vi "ModeEditMain.vi"(0 "当前零件序号":i32) -> (1 "ModelEditInfo":T2, 2 "产品程式设定OK":bool)   [LabVIEW 2014]
uses:
  Global.vi
  <vilib>/Utility/file.llb/Write To Spreadsheet File (I64).vi
  ModeEditeControl.ctl
  ModelInfo.ctl
  Controls/XYZRPos.ctl
panel:
  in  "托盘1螺丝型号":T1=enum."一字螺丝M2.5*8"
  in  "Btn_添加点位":bool
  in  "Btn_删除点位":bool
  in  "退出按钮":bool
  in  "选项卡控件":enum32{"产品程式维护", "锁螺丝点位维护", "点位示意图", "拧紧程式参数维护"}(tab)
  out "已建立产品程式信息":string[][](table)=[["产品型号1", "0", "5", "6", "E:\\771半自动装配系统-2019200427\\Model\\产品型号1\\产品型号1_CAD点位坐标.txt", "0", "0", "0", "0", "0", "0", "0", "1", "92", "93", "93", "94", "95", "94", "97", "94", "92", "93", "18500", "18500"]]
  out "提示信息":string
  in  "Btn_添加新产品程式":bool
  in  "Btn_删除产品程式":bool
  in  "Btn_更新产品程式信息":bool
  in  "产品信息":T3
  in  "Btn_PCB2~4锁螺丝时机械手角度，取料托盘号与PCB1相同":bool
  out "Mark拍照点坐标":T4[](array[typedef])
  in  "Btn_读取Mark1&Mark2(P21 P22)坐标":bool
  in  "Btn_根据第1组Mark点计算PCB1其它拍照点坐标":bool
  in  "读取CAD文档点位信息":bool
  in  "Btn_更新点位信息表":bool
  out "实际点位示意图":T6(plugin-control)
  out "CAD图纸点位示意图":T6(plugin-control)
  in  "Btn_删除拧紧程式参数":bool
  in  "Btn_更新拧紧程式参数":bool
  in  "拧紧程式参数表":string[][](table)=[["92", "2", "3", "4", "6", "7", "8", "9"], ["93", "12", "13", "14", "16", "17", "18", "19"], ["94", "22", "23", "24", "26", "27", "28", "29"], ["95", "32", "33", "34", "36", "37", "38", "39"]]
  out "不同型号螺丝放料点与拍照点高度差":string[][](table)=[["一字螺丝M2.5*4"], ["一字螺丝M2.5*6"], ["一字螺丝M2.5*8"], ["一字螺丝M2.5*10"], ["一字螺丝M2.5*12"], ["一字螺丝M2.5*14"], ["一字螺丝M2.5*16"], ["一字螺丝M2.5*18"], ["一字螺丝M2.5*20"], ["一字螺丝M3*4"], ["一字螺丝M3*6"], ["一字螺丝M3*8"], ["一字螺丝M3*10"], ["一字螺丝M3*12"], ["一字螺丝M3*14"], ["一字螺丝M3*16"], ["一字螺丝M3*18"], ["一字螺丝M3*20"], ["一字螺丝M4*6"], ["一字螺丝M4*8"], ["一字螺丝M4*10"], ["一字螺丝M4*12"], ["一字螺丝M4*14"], ["一字螺丝M4*16"], ["一字螺丝M4*18"], ["一字螺丝M4*20"], ["十字螺丝M2.5*4"], ["十字螺丝M2.5*6"], ["十字螺丝M2.5*8"], ["十字螺丝M2.5*10"], ["十字螺丝M2.5*12"], ["十字螺丝M2.5*14"], ["十字螺丝M2.5*16"], ["十字螺丝M2.5*18"], ["十字螺丝M2.5*20"], ["十字螺丝M3*4"], ["十字螺丝M3*6"], ["十字螺丝M3*8"], ["十字螺丝M3*10"], ["十字螺丝M3*12"], ["十字螺丝M3*14"], ["十字螺丝M3*16"], ["十字螺丝M3*18"], ["十字螺丝M3*20"], ["十字螺丝M4*6"], ["十字螺丝M4*8"], ["十字螺丝M4*10"], ["十字螺丝M4*12"], ["十字螺丝M4*14"], ["十字螺丝M4*16"], ["十字螺丝M4*18"], ["十字螺丝M4*20"]]
  # "白色代表自动锁螺丝，灰色不锁"
  # "白色代表自动锁螺丝，灰色不锁"
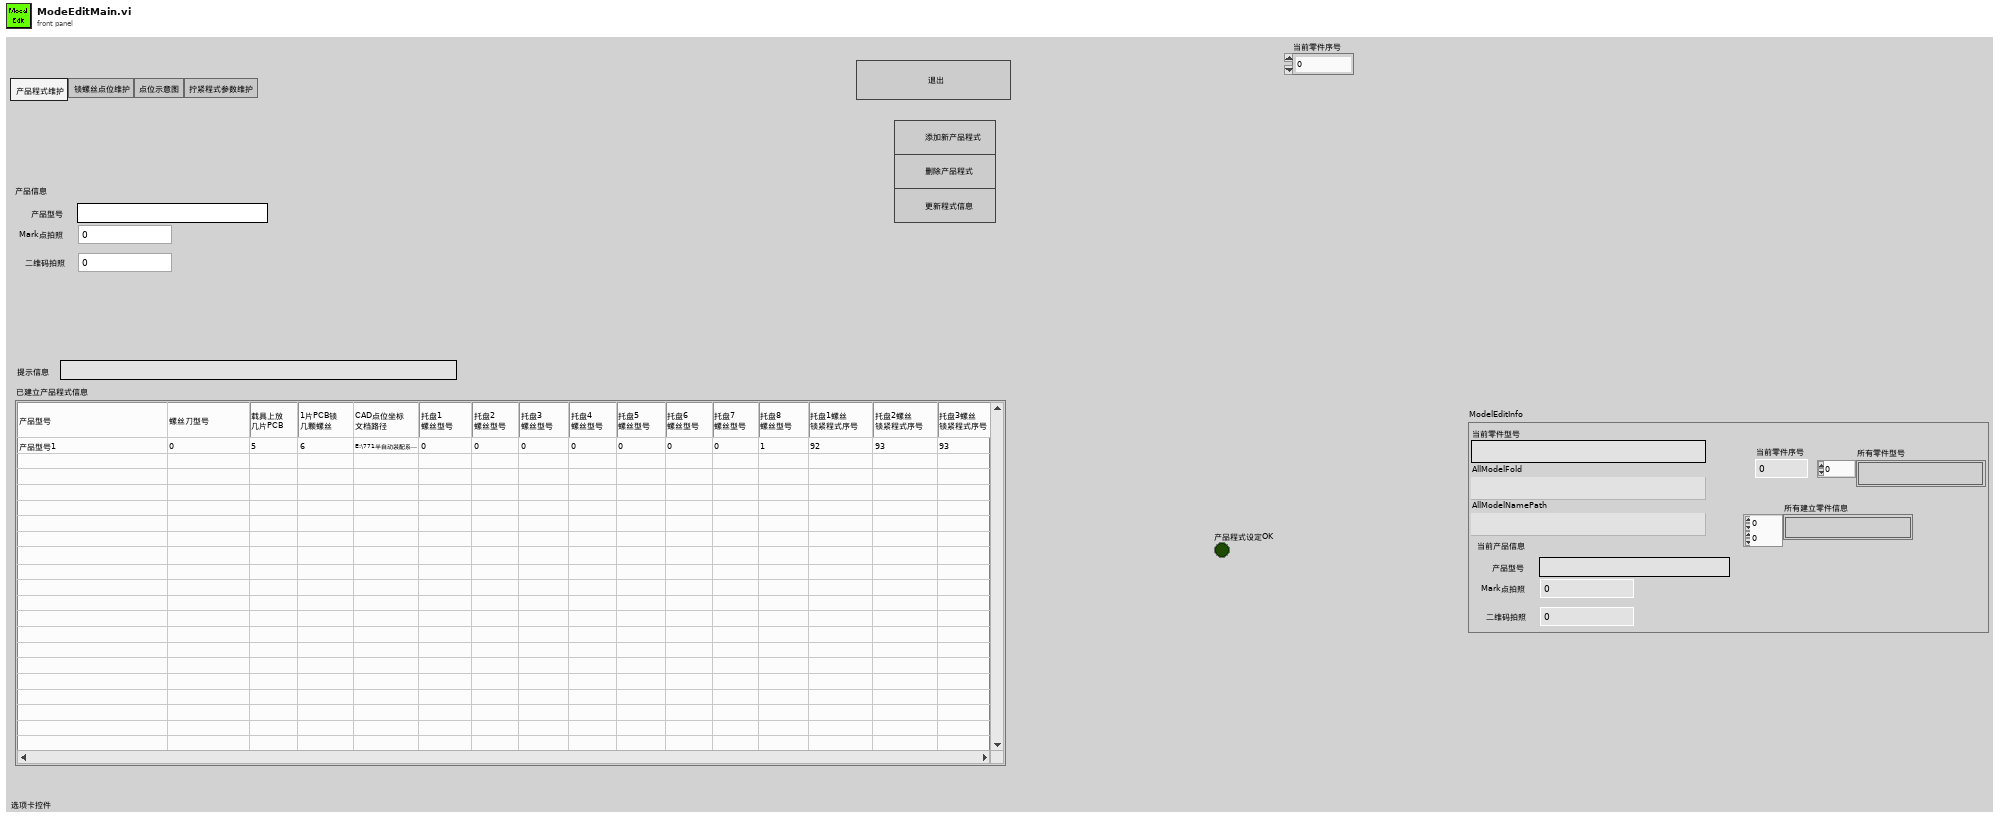
[diagram p1: front panel]
types:
  T1 = typedef "控件-螺丝型号.ctl" = enum16{"不供料", "一字螺丝M2.5*4", "一字螺丝M2.5*6", "一字螺丝M2.5*8", "一字螺丝M2.5*10", "一字螺丝M2.5*12", "一字螺丝M2.5*14", "一字螺丝M2.5*16", "一字螺丝M2.5*18", "一字螺丝M2.5*20", "一字螺丝M3*4", "一字螺丝M3*6", "一字螺丝M3*8", "一字螺丝M3*10", "一字螺丝M3*12", "一字螺丝M3*14", "一字螺丝M3*16", "一字螺丝M3*18", "一字螺丝M3*20", "一字螺丝M4*6", "一字螺丝M4*8", "一字螺丝M4*10", "一字螺丝M4*12", "一字螺丝M4*14", "一字螺丝M4*16", "一字螺丝M4*18", "一字螺丝M4*20", "十字螺丝M2.5*4", "十字螺丝M2.5*6", "十字螺丝M2.5*8", "十字螺丝M2.5*10", "十字螺丝M2.5*12", "十字螺丝M2.5*14", "十字螺丝M2.5*16", "十字螺丝M2.5*18", "十字螺丝M2.5*20", "十字螺丝M3*4", "十字螺丝M3*6", "十字螺丝M3*8", "十字螺丝M3*10", "十字螺丝M3*12", "十字螺丝M3*14", "十字螺丝M3*16", "十字螺丝M3*18", "十字螺丝M3*20", "十字螺丝M4*6", "十字螺丝M4*8", "十字螺丝M4*10", "十字螺丝M4*12", "十字螺丝M4*14", "十字螺丝M4*16", "十字螺丝M4*18", "十字螺丝M4*20"}
  T2 = typedef "ModeEditeControl.ctl" = cluster{"AllModelFold":path, "AllModelNamePath":path, "所有零件型号":string[], "当前零件型号":string, "所有建立零件信息":string[][], "当前零件序号":i32, "当前产品信息":T3}
  T3 = typedef "ModelInfo.ctl" = cluster{"产品型号":string, "二维码拍照":u32, "Mark点拍照":u32}
  T4 = typedef "XYZRPos+左右手.ctl" = cluster{"坐标":T5, "左右手":dbl}
  T5 = typedef "XYZRPos.ctl" = cluster{"X":dbl, "Y":dbl, "Z":dbl, "R":dbl}
  T6 = typedef "IMAQ Image.ctl" = refnum<image>
  T7 = typedef "控件-点位示意图动作.ctl" = enum16{"初始化点位示意图", "更新点位示意图"}
  T8 = cluster{"CAD图纸点位示意图":refnum<vi>, "实际点位示意图":refnum<vi>}
  T9 = typedef "ModeEditeControl.ctl" = cluster{"Root":path, "AllModelFold":path, "AllModelNamePath":path, "所有零件型号":string[], "当前零件型号":string, "所有建立零件信息":string[][], "当前零件序号":i32, "当前产品所有点位信息":cluster{"当前点位序号":i32, "点位信息路径":path, "CAD点位坐标路径":path, "点位信息表":string[][], "当前点位信息":T10, "CAD图纸点位个数":i32}, "当前产品信息":T13, "所有螺丝和垫片型号Path":path, "Mark拍照点坐标":T4[][], "自动锁螺丝: PCB孔拍照点-多片PCB(去除未勾选的)":T4[], "8个供料盘是否供料-1PCB(去除未勾选的)":bool[], "8个供料盘是否拍照取料":bool[], "自动锁螺丝: 1PCB每颗螺丝来自哪个供料盘U8(去除未勾选的)":u8[], "自动锁螺丝: 1PCB每颗螺丝拧紧程式编号U8(去除未勾选的)":u8[], "4个预锁程式+4个复锁程式编号U8":u8[], "自动锁螺丝: 锁螺丝相对拍照时旋转角度-多片PCB(去除未勾选的)":i32[], "自动锁螺丝: 点位补偿值-多片PCB(去除未勾选的)":T11[], "1PCB上自动锁螺丝个数(去除未勾选的)":i32, "自动锁螺丝: 放料点相对拍照点高度差-多片PCB(去除未勾选的)":dbl[], "8个供料盘是否供料(包括未勾选的)":bool[], "已勾选的自动锁螺丝点位供料盘设定错误":bool, "自动锁螺丝: 复锁拍照点-多片PCB(去除未勾选的)":T4[][], "自动锁螺丝: 1PCB每颗螺丝外径*10(去除未勾选的)":u32[], "拧紧程式参数":cluster{"所有拧紧程式参数表路径":path, "所有拧紧程式参数表":string[][], "自动锁螺丝: 每个托盘螺丝拧紧程式参数":T15[], "自动锁螺丝: 预锁复锁拧紧程式参数":T15[], "所有拧紧程式参数表当前行":i32}, "已勾选的自动锁螺丝点位拧紧程式序号设定错误":bool}
  T10 = typedef "锁附点位信息.ctl" = cluster{"点位名称":string, "点位坐标(图纸)":T11, "点位坐标(实际)":T5, "补偿值":T11, "锁附时机械手角度":T12, "放料点相对Mark\n拍照点高度差":dbl, "选择螺丝托盘":enum32{"托盘1", "托盘2", "托盘3", "托盘4", "托盘5", "托盘6", "托盘7", "托盘8"}, "拧紧程式序号":u16, "预锁程式序号":u16, "复锁程式序号":u16, "自动锁螺丝":bool}
  T11 = typedef "XYZPos.ctl" = cluster{"X":dbl, "Y":dbl, "Z":dbl}
  T12 = typedef "锁附时机械手角度.ctl" = enum16{"0度", "顺时针90度", "顺时针180度", "逆时针90度", "逆时针180度"}
  T13 = typedef "ModelInfo.ctl" = cluster{"产品型号":string, "螺丝刀型号":T14, "载具上放几片PCB":u16, "1片PCB锁几颗螺丝":u16, "CAD点位坐标文档路径":path, "托盘1螺丝型号":T1, "托盘2螺丝型号":T1, "托盘3螺丝型号":T1, "托盘4螺丝型号":T1, "托盘5螺丝型号":T1, "托盘6螺丝型号":T1, "托盘7螺丝型号":T1, "托盘8螺丝型号":T1, "托盘1螺丝锁紧程式序号":u32, "托盘2螺丝锁紧程式序号":u32, "托盘3螺丝锁紧程式序号":u32, "托盘4螺丝锁紧程式序号":u32, "托盘5螺丝锁紧程式序号":u32, "托盘6螺丝锁紧程式序号":u32, "托盘7螺丝锁紧程式序号":u32, "托盘8螺丝锁紧程式序号":u32, "预锁程式序号":u32, "复锁程式序号":u32, "复锁拍照点与Mark拍照点高度差":dbl, "取料点与P2高度差":dbl, "拍PCB孔曝光时间":u32, "取料拍螺帽曝光时间":u32, "复锁拍螺帽曝光时间":u32, "下相机曝光时间":u32}
  T14 = typedef "螺丝刀类型.ctl" = enum16{"螺丝刀1-1*3mm", "螺丝刀2-1.5*3mm", "螺丝刀3-2*3mm", "螺丝刀4-2*4mm", "螺丝刀5-2.5*4mm"}
  T15 = typedef "控件-拧紧程式参数.ctl" = cluster{"螺距":dbl, "入牙段转速":dbl, "入牙段转角":dbl, "快速段转速":dbl, "快速段转角":dbl, "快速段Z补偿":dbl, "拧紧转速":dbl}
  T16 = typedef "欧姆龙PLC Action.ctl" = enum16{"读设备状态", "初始化", "待命", "重新初始化", "读触发信息", "读第1组Mark点坐标", "读第2组Mark点坐标", "写基本信息", "写第1组Mark点坐标", "写第2组Mark点坐标", "写相机中心到出线头的距离", "写一笔轨迹到PLC", "写入进线前段点位", "写入板内布线点位", "写入出线布线点位", "写入数据写入完成信号", "获取信息", "写入进出线方向", "写加工信号"}
  T17 = typedef "欧姆龙PLC Action.ctl" = enum16{"初始化", "重新初始化", "读触发信息", "读示教坐标P1P2", "读示教坐标P3P4", "读示教坐标P11P12", "读示教坐标P13P14", "读第1组Mark点坐标", "读第2组Mark点坐标", "读第3组Mark点坐标", "自检：写螺丝刀拍照结果和Finish", "自检：写供料盘二维码拍照结果和Finish", "读第4组Mark点坐标", "写取料点相对拍照点移动量", "写放料点坐标", "写放螺丝时相对当前拍照点偏移量", "写取料点相对拍照点移动量&放料点坐标", "写螺杆拍照完成Finish", "写读取锁附结果完成信号", "写复锁时相对拍照点移动量", "写数据-测试用", "写当前产品基本供料信息", "写当前产品每颗螺丝来自哪个供料盘", "写当前产品每颗螺丝拧紧程式序号", "写当前产品4个预锁程式和4个复锁程式序号", "写第1组Mark点坐标", "写第2组Mark点坐标", "写第3组Mark点坐标", "写第4组Mark点坐标", "写夹螺杆点到拍螺帽点距离", "写第1组复锁拍照点", "写第2组复锁拍照点", "写第3组复锁拍照点", "写第4组复锁拍照点", "写启用的托盘螺丝拧紧程式参数", "写预锁复锁拧紧程式参数", "获取信息"}
  T18 = enum16{"计算PCB1其它拍照点坐标", "计算PCB2其它拍照点坐标", "计算PCB3其它拍照点坐标", "计算PCB4其它拍照点坐标"}
  T19 = typedef "LVRowAndColumnTypeDef.ctl" = cluster{"Row":i32, "Column":i32}
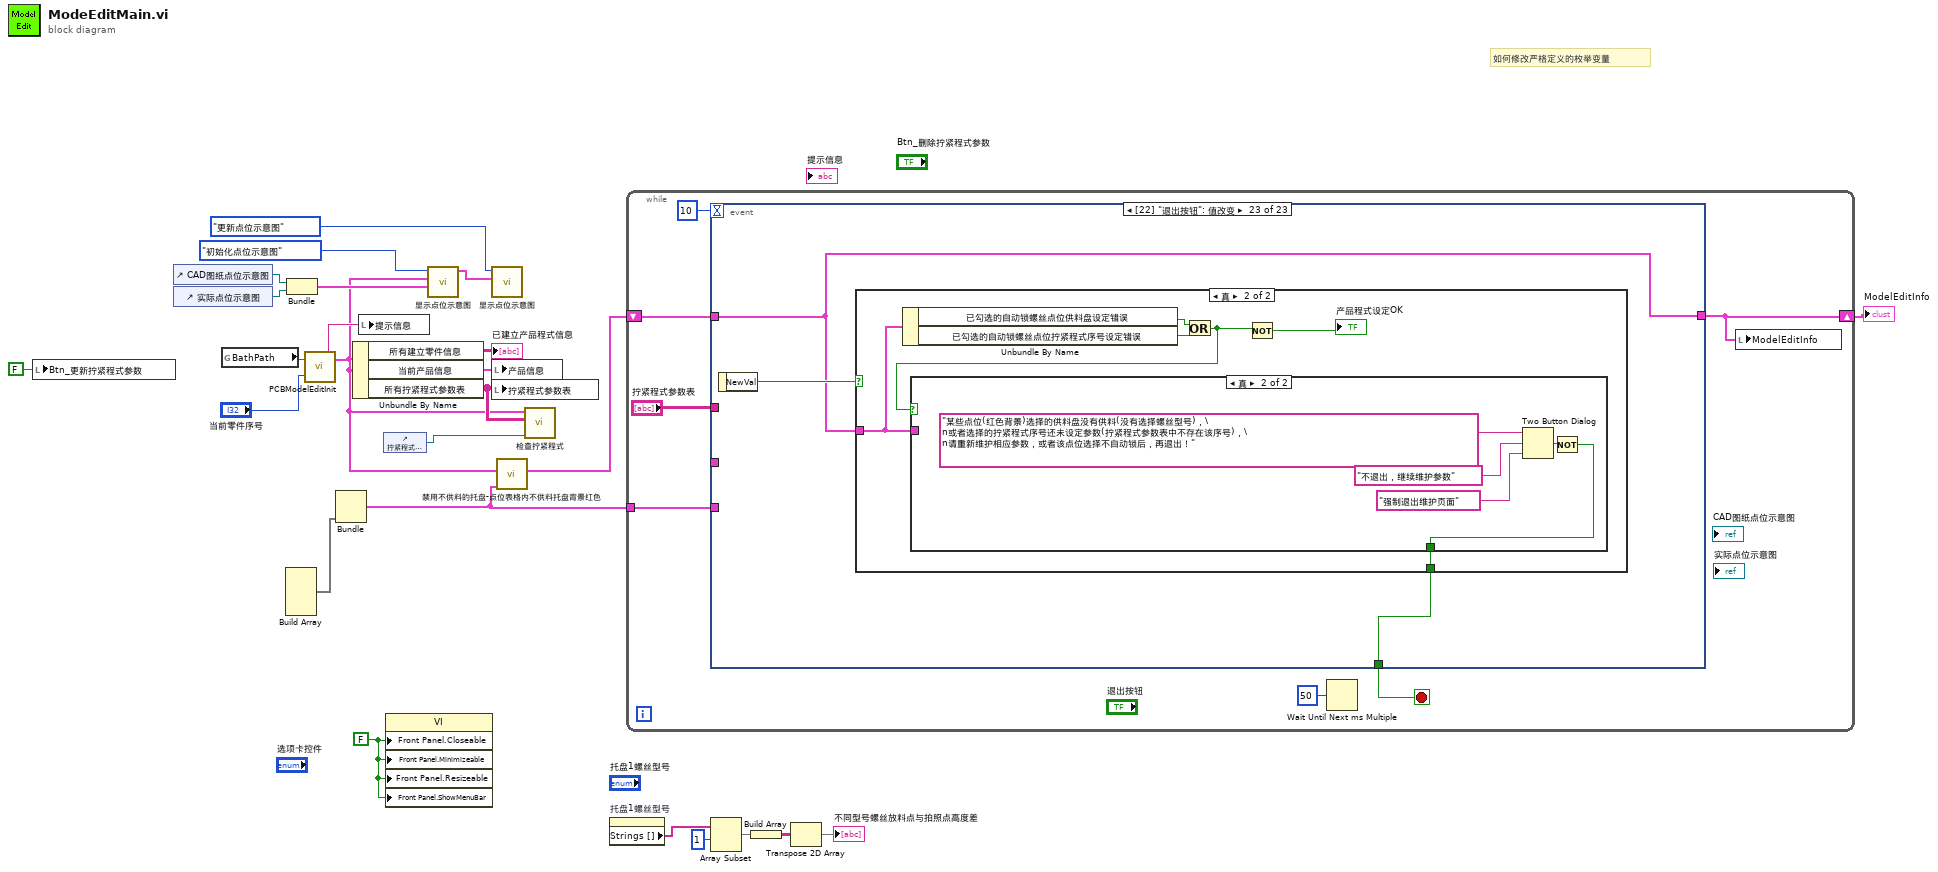
[diagram p0: block diagram]
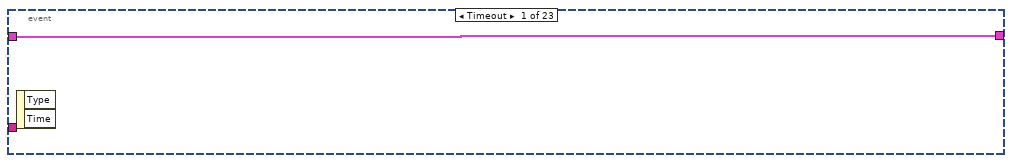
[diagram p2: hidden frame]
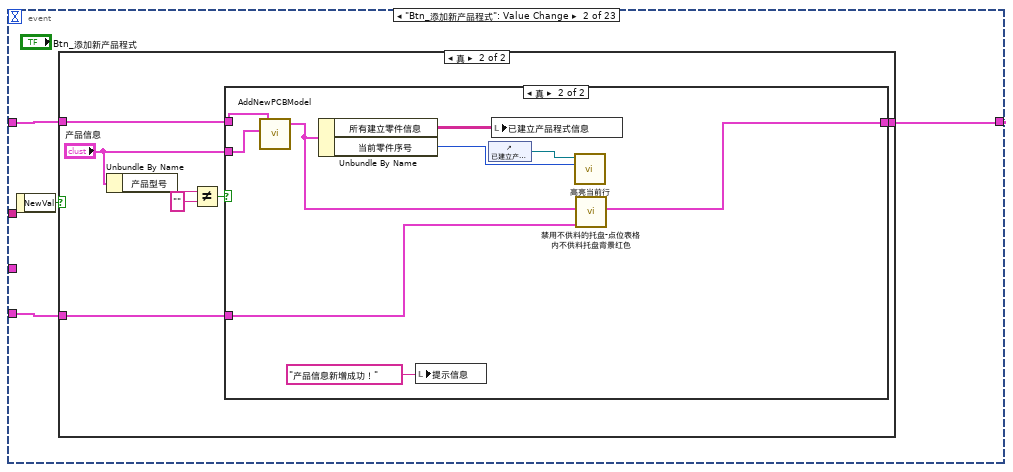
[diagram p3: hidden frame]
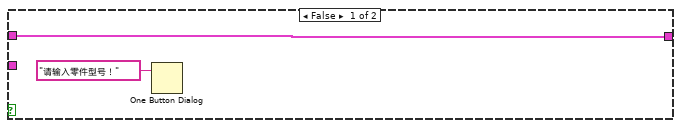
[diagram p5: hidden frame]
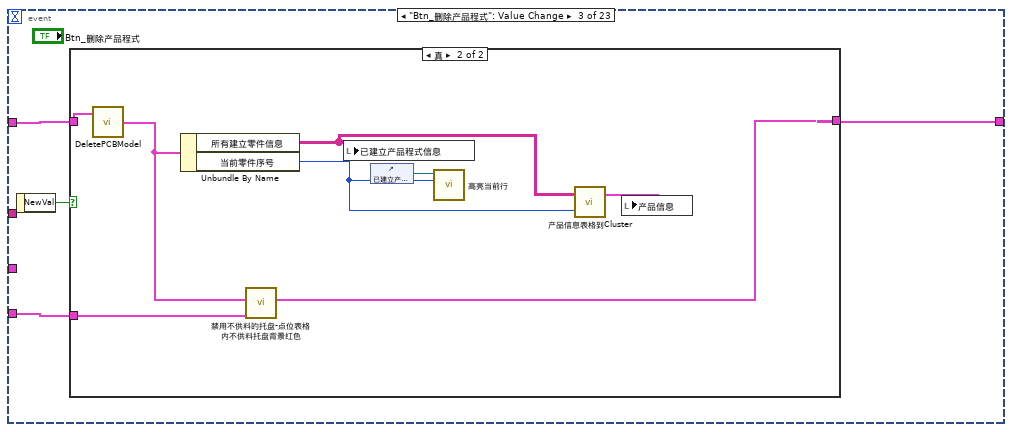
[diagram p6: hidden frame]
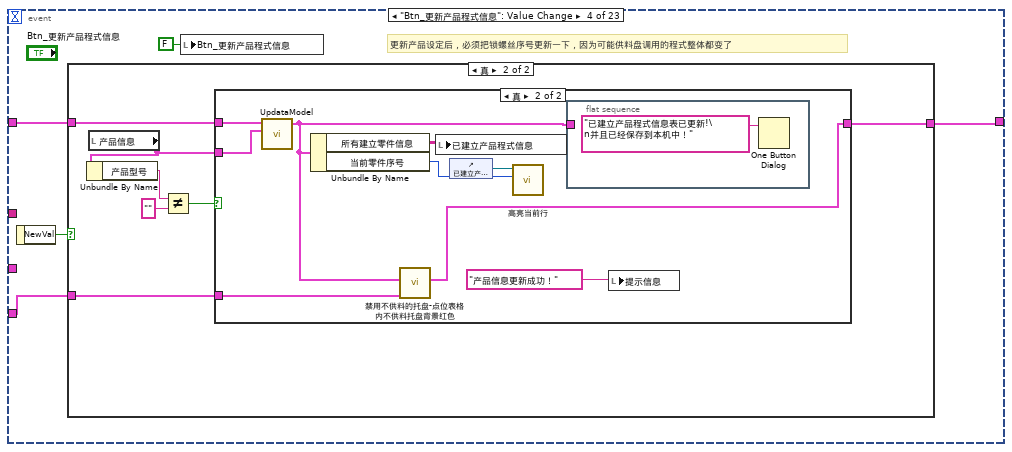
[diagram p8: hidden frame]
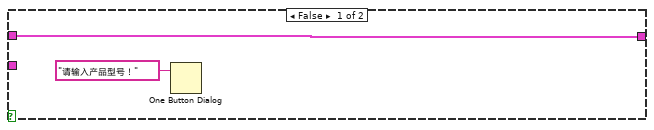
[diagram p10: hidden frame]
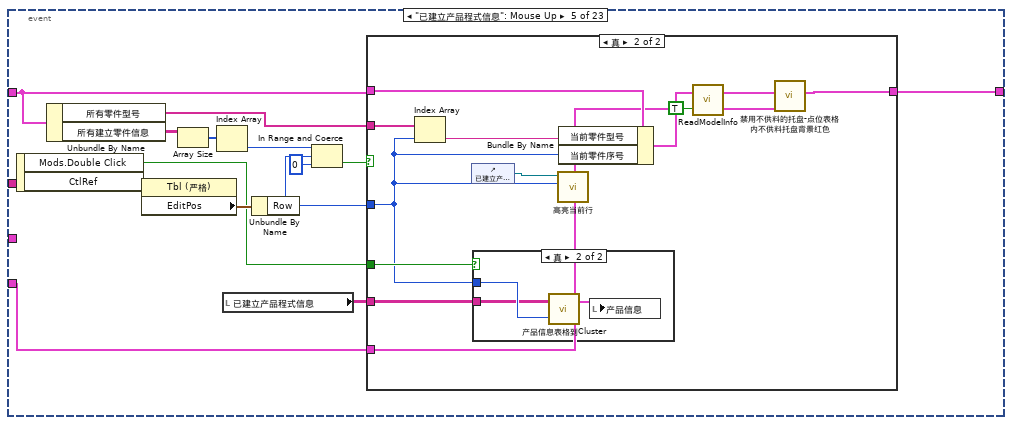
[diagram p11: hidden frame]
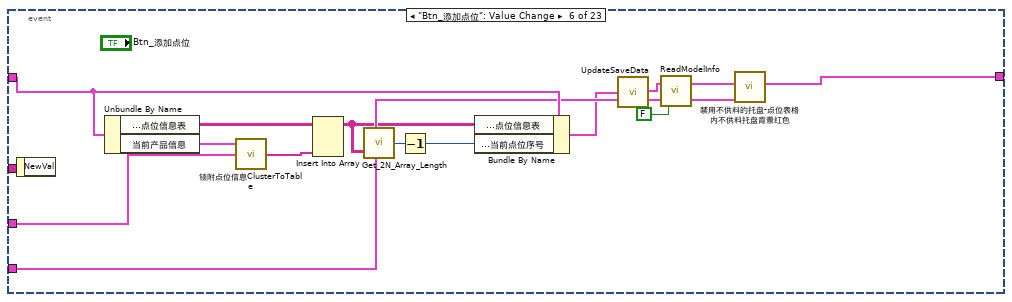
[diagram p14: hidden frame]
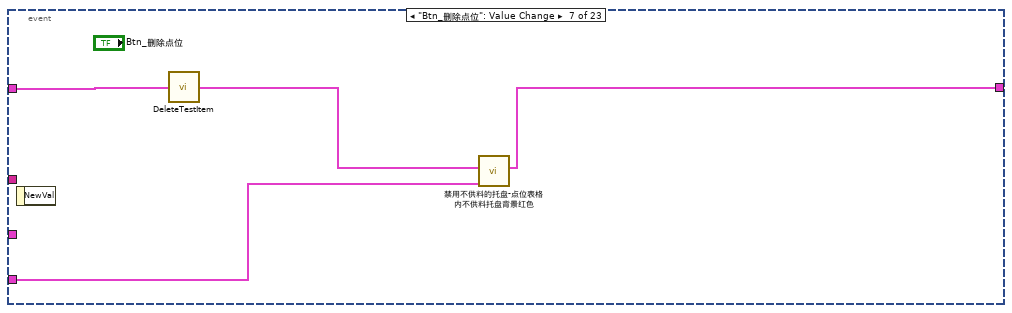
[diagram p15: hidden frame]
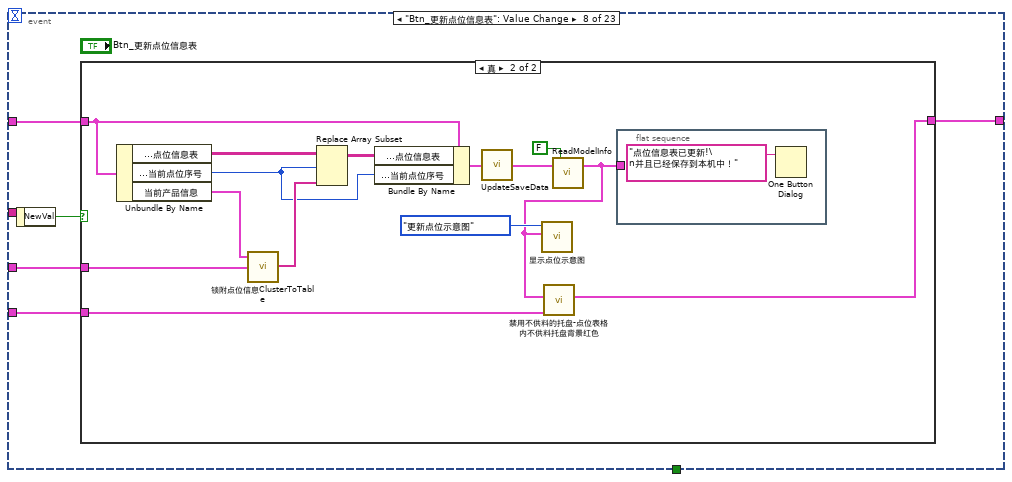
[diagram p16: hidden frame]
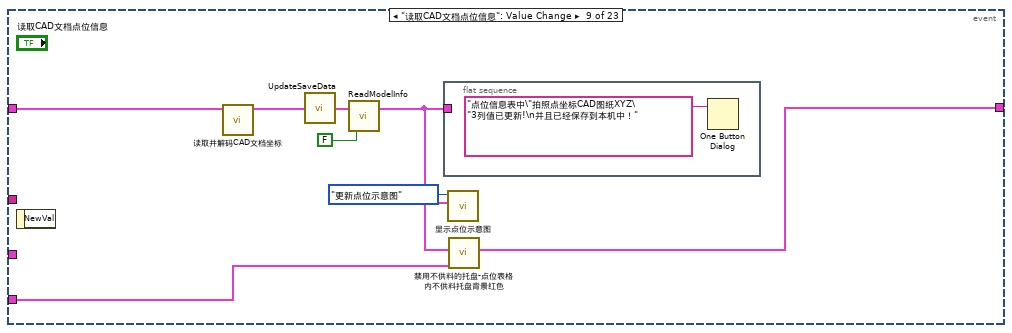
[diagram p18: hidden frame]
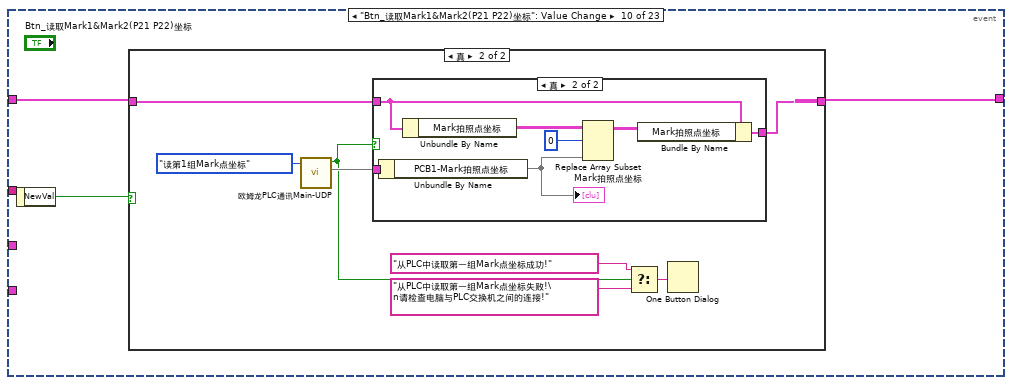
[diagram p19: hidden frame]
diagram:
  w30 = FALSE ("Front Panel Window:Closeable")
  # "如何修改严格定义的枚举变量"
  n1 = local write "Btn_更新拧紧程式参数"(FALSE ("Btn_更新拧紧程式参数")) -> ()
  n2 = control-ref of="CAD图纸点位示意图"() -> (w25:refnum<vi>)
  n3 = control-ref of="实际点位示意图"() -> (w24:refnum<vi>)
  n4 = global read "Global.vi" "BathPath"() -> (w32:path)
  n5 = Build Array() -> (w13:void[], w19:dbl, w18:dbl, w17:dbl, w16:dbl, w15:dbl, w14:dbl)
  n6 = Bundle("CAD图纸点位示意图"=w25, "实际点位示意图"=w24) -> (w23:T8)  [unwired: 1 in]
  n7 = call "PCBModelEditInit.vi"("当前零件序号"="当前零件序号", "path"=w32) -> ("Msg"=w31:string, "ModelEditInfo"=w2:T2)
  n8 = Bundle(w13) -> (w11:cluster{void, void, void, void[]}, w12, w27)  [unwired: 2 in]
  n9 = Unbundle By Name(w2) -> ("所有建立零件信息"=→"已建立产品程式信息":string[][], "当前产品信息"=w26:T3, "所有拧紧程式参数表"=w3:string[][])
  n10 = local write "提示信息"(w31) -> ()
  n11 = control-ref of="拧紧程式参数表"() -> (w1:refnum<vi>)
  n12 = property class="VI"("Front Panel.Closeable"=w30, "Front Panel.Minimizeable"=w30, "Front Panel.Resizeable"=w30, "Front Panel.ShowMenuBar"=w30) -> ()  [unwired: 2 in, 2 out]
  n13 = call "显示点位示意图.vi"("Img引用Cluster"=w23, "ModelEditInfo"=w2, "显示点位动作"=控件-点位示意图动作."初始化点位示意图") -> ("ModelEditInfo out"=w20:T2)  [unwired: 8 in]
  n14 = call "显示点位示意图.vi"("ModelEditInfo"=w20, "显示点位动作"=控件-点位示意图动作."更新点位示意图") -> ()  [unwired: 9 in, 1 out]
  n15 = local write "产品信息"(w26) -> ()
  n16 = local write "拧紧程式参数表"(w3) -> ()
  n17 = call "禁用不供料的托盘-点位表格内不供料托盘背景红色.vi"("引用Cluster"=w11, "ModelEditInfo in"=w2) -> ("ModelEditInfo out"=w10:T9)  [unwired: 8 in, 1 out]
  n18 = call "检查拧紧程式.vi"("拧紧程式参数表引用"=w1, "拧紧程式参数表输入"=w3, "ModelEditInfo"=w2) -> ()  [unwired: 7 in, 2 out]
  n19 = property on="托盘1螺丝型号" class="Enum (严格)"() -> ("Strings []"=w9:string[])  [unwired: 2 in, 2 out]
  n20 = while {
    shift-right: [w36] -> w33
    shift-left: w10 -> [w39]
    tunnel: w11 -> [w35]
    stop <- w38 stop-if-true
    n21 = event shown="[22] \"退出按钮\": 值改变" {
      selector: _ -> [_ _ _ _ _ _ _ _ _ _ _ _ _ _ _ _ _ _ _ _ _ _ _]
      dyn-events: _ -> [_ _ _ _ _ _ _ _ _ _ _ _ _ _ _ _ _ _ _ _ _ _ _]
      timeout: 10 -> [_ _ _ _ _ _ _ _ _ _ _ _ _ _ _ _ _ _ _ _ _ _ _]
      tunnel: w39 -> [w42 w45 w68 w83 w109 w145 w151 w155 w180 w184 w203 w224 w244 w270 w278 w288 w298 w308 w315 w341 w379 w383 w400]
      tunnel: [w42 w44 w67 w82 w108 w134 w148 w153 w173 w182 w202 w222 w242 w262 w272 w283 w292 w302 w314 w346 w373 w386 w400] -> w36
      tunnel: [_ _ _ _ _ _ _ _ _ _ _ _ _ _ _ _ _ _ _ _ _ _ w401] -> w38
      tunnel: [_ _ _ _ _ w144 _ w154 _ _ _ _ _ _ _ _ _ _ _ _ _ _ _] -> w37
      tunnel: w35 -> [_ w43 w66 w79 w104 w141 w149 w152 w176 _ _ _ _ w265 w275 w286 w296 w304 w310 w345 w372 _ _]
      tunnel: "拧紧程式参数表" -> [_ _ _ _ _ _ _ _ _ _ _ _ _ _ _ _ _ _ _ w342 _ _ _]
      event Timeout {
        n22 = event-data() -> ()  [unwired: 1 in, 2 out]
      }
      event "Btn_添加新产品程式": Value Change {
        n23 = event-data() -> ("NewVal"=w46:bool)  [unwired: 1 in]
        n24 = case shown="真" w46 {
          tunnel: w45 -> [w47 w51]
          tunnel: [w47 w52] -> w44
          tunnel: w43 -> [_ w48]
          frame False {
          }
          frame True {
            n25 = Unbundle By Name("产品信息") -> ("产品型号"=w50:string)
            n26 = Not Equal?(x=w50, y="") -> (x != y?=w53:bool)
            n27 = case shown="真" w53 {
              tunnel: w51 -> [w55 w65]
              tunnel: [w55 w57] -> w52
              tunnel: "产品信息" -> [_ w62]
              tunnel: w48 -> [_ w58]
              frame False {
                n28 = One Button Dialog(message="请输入零件型号！") -> ()  [unwired: 1 in, 1 out]
              }
              frame True {
                n29 = call "AddNewPCBModel.vi"("新增零件信息"=w62, "ModelEditInfo in"=w65) -> ("ModelEditInfo out"=w59:T2)  [unwired: 4 in]
                n30 = Unbundle By Name(w59) -> ("所有建立零件信息"=w63:string[][], "当前零件序号"=w60:i32)
                n31 = local write "提示信息"("产品信息新增成功！" ("ReadGerberMsg")) -> ()
                n32 = control-ref of="已建立产品程式信息"() -> (w61:refnum<vi>)
                n33 = local write "已建立产品程式信息"(w63) -> ()
                n34 = call "高亮当前行.vi"("Row"=w60, "Table输入"=w61) -> ()  [unwired: 9 in, 1 out]
                n35 = call "禁用不供料的托盘-点位表格内不供料托盘背景红色.vi"("引用Cluster"=w58, "ModelEditInfo in"=w59) -> ("ModelEditInfo out"=w57:T9)  [unwired: 8 in, 1 out]
              }
            }
          }
        }
      }
      event "Btn_删除产品程式": Value Change {
        n36 = event-data() -> ("NewVal"=w69:bool)  [unwired: 1 in]
        n37 = case shown="真" w69 {
          tunnel: w68 -> [w70 w78]
          tunnel: [w70 w71] -> w67
          tunnel: w66 -> [_ w72]
          frame False {
          }
          frame True {
            n38 = call "DeletePCBModel.vi"("ModelEditInfo in"=w78) -> ("ModelEditInfo out"=w73:T2)
            n39 = Unbundle By Name(w73) -> ("所有建立零件信息"=w75:string[][], "当前零件序号"=w76:i32)
            n40 = call "禁用不供料的托盘-点位表格内不供料托盘背景红色.vi"("引用Cluster"=w72, "ModelEditInfo in"=w73) -> ("ModelEditInfo out"=w71:T9)  [unwired: 8 in, 1 out]
            n41 = local write "已建立产品程式信息"(w75) -> ()
            n42 = control-ref of="已建立产品程式信息"() -> (w77:refnum<vi>)
            n43 = call "高亮当前行.vi"("Row"=w76, "Table输入"=w77) -> ()  [unwired: 9 in, 1 out]
            n44 = call "产品信息表格到Cluster.vi"("Row"=w76, "已建立量测零件信息"=w75) -> ("零件信息"=w74:T13)
            n45 = local write "产品信息"(w74) -> ()
          }
        }
      }
      event "Btn_更新产品程式信息": Value Change {
        # "更新产品设定后，必须把锁螺丝序号更新一下，因为可能供料盘调用的程式整体都变了"
        n46 = event-data() -> ("NewVal"=w81:bool)  [unwired: 1 in]
        n47 = case shown="真" w81 {
          tunnel: w83 -> [w84 w88]
          tunnel: [w84 w87] -> w82
          tunnel: w79 -> [_ w85]
          frame False {
          }
          frame True {
            n48 = local read "产品信息"() -> (w86:T3)
            n49 = Unbundle By Name(w86) -> ("产品型号"=w89:string)
            n50 = Not Equal?(x=w89, y="") -> (x != y?=w90:bool)
            n51 = case shown="真" w90 {
              tunnel: w88 -> [w92 w100]
              tunnel: [w92 w94] -> w87
              tunnel: w86 -> [_ w99]
              tunnel: w85 -> [_ w96]
              frame False {
                n52 = One Button Dialog(message="请输入产品型号！") -> ()  [unwired: 1 in, 1 out]
              }
              frame True {
                n53 = call "UpdataModel.vi"("更新零件信息"=w99, "ModelEditInfo in"=w100) -> ("ModelEditInfo out"=w95:T2)  [unwired: 4 in]
                n54 = Unbundle By Name(w95) -> ("所有建立零件信息"=w102:string[][], "当前零件序号"=w97:i32)
                n55 = call "禁用不供料的托盘-点位表格内不供料托盘背景红色.vi"("引用Cluster"=w96, "ModelEditInfo in"=w95) -> ("ModelEditInfo out"=w94:T9)  [unwired: 8 in, 1 out]
                n56 = local write "已建立产品程式信息"(w102) -> ()
                n57 = control-ref of="已建立产品程式信息"() -> (w98:refnum<vi>)
                n58 = call "高亮当前行.vi"("Row"=w97, "Table输入"=w98) -> ()  [unwired: 9 in, 1 out]
                n59 = flat-sequence {
                  tunnel: w95 -> [_]
                  frame #0 {
                    n60 = One Button Dialog(message="已建立产品程式信息表已更新!\n并且已经保存到本机中！" ("消息")) -> ()  [unwired: 1 in, 1 out]
                  }
                }
                n61 = local write "提示信息"("产品信息更新成功！" ("ReadGerberMsg")) -> ()
              }
            }
          }
        }
        n62 = local write "Btn_更新产品程式信息"(FALSE ("Btn_更新量测信息")) -> ()
      }
      event "已建立产品程式信息": Mouse Up {
        n63 = event-data() -> ("Mods.Double Click"=w106:bool, "CtlRef"=w116:refnum<vi>)  [unwired: 1 in]
        n64 = Unbundle By Name(w109) -> ("所有零件型号"=w107:string[], "所有建立零件信息"=w115:string[][])
        n65 = property class="Tbl (严格)"(reference=w116) -> ("EditPos"=w117:T19)  [unwired: 1 in, 2 out]
        n66 = Array Size(array=w115) -> (size(s)=w114:i32[])
        n67 = Index Array(array=w114) -> (element=w110:i32)  [unwired: 1 in]
        n68 = local read "已建立产品程式信息"() -> (w105:string[][])
        n69 = Unbundle By Name(w117) -> ("Row"=w113:i32)
        n70 = In Range and Coerce(upper limit=w110, x=w113, lower limit=0 ("下限")) -> (In Range?=w112:bool)  [unwired: 1 out]
        n71 = case shown="真" w112 {
          tunnel: w113 -> [_ w123]
          tunnel: w109 -> [w118 w130]
          tunnel: [w118 w119] -> w108
          tunnel: w107 -> [_ w127]
          tunnel: w106 -> [_ w126]
          tunnel: w105 -> [_ w125]
          tunnel: w104 -> [_ w120]
          frame False {
          }
          frame True {
            n72 = Index Array(array=w127, index=w123) -> (element=w129:string)
            n73 = control-ref of="已建立产品程式信息"() -> (w124:refnum<vi>)
            n74 = case shown="真" w126 {
              tunnel: w123 -> [_ w132]
              tunnel: w125 -> [_ w131]
              frame False {
              }
              frame True {
                n75 = call "产品信息表格到Cluster.vi"("Row"=w132, "已建立量测零件信息"=w131) -> ("零件信息"=w133:T13)
                n76 = local write "产品信息"(w133) -> ()
              }
            }
            n77 = call "高亮当前行.vi"("Row"=w123, "Table输入"=w124) -> ()  [unwired: 9 in, 1 out]
            n78 = Bundle By Name(cluster=w130, "当前零件型号"=w129, "当前零件序号"=w123) -> (w128:T9)
            n79 = call "ReadModelInfo.vi"("更新量测项目序号"=TRUE, "ModelEditInfo in"=w128) -> ("ModelEditInfo out"=w121:T2)  [unwired: 1 in]
            n80 = call "禁用不供料的托盘-点位表格内不供料托盘背景红色.vi"("引用Cluster"=w120, "ModelEditInfo in"=w121) -> ("ModelEditInfo out"=w119:T9)  [unwired: 8 in, 1 out]
          }
        }
      }
      event "Btn_添加点位": Value Change {
        n81 = event-data() -> ()  [unwired: 1 in, 1 out]
        n82 = Unbundle By Name(w145) -> ("当前产品所有点位信息.点位信息表"=w146:string[][], "当前产品信息"=w142:T13)
        n83 = call "锁附点位信息ClusterToTable.vi"("锁附点位信息"=w144, "当前产品信息"=w142) -> ("点位信息表格一行"=w147:string[])  [unwired: 1 in]
        n84 = Insert Into Array ("数组插入")(array=w146, new element=w147) -> (w137:string[][])  [unwired: 2 in]
        n85 = call "Get_2N_Array_Length.vi"("StringArray"=w137) -> ("Numeric"=w139:i32)  [unwired: 1 in]
        n86 = Decrement(x=w139) -> (x-1=w135:i32)
        n87 = Bundle By Name(cluster=w145, "当前产品所有点位信息.点位信息表"=w137, "当前产品所有点位信息.当前点位序号"=w135) -> (w140:T9)
        n88 = call "UpdateSaveData.vi"("ModelEditInfo in"=w140) -> ("ModelEditInfo out"=w138:T2)
        n89 = call "ReadModelInfo.vi"("更新量测项目序号"=FALSE, "ModelEditInfo in"=w138) -> ("ModelEditInfo out"=w143:T2)  [unwired: 1 in]
        n90 = call "禁用不供料的托盘-点位表格内不供料托盘背景红色.vi"("引用Cluster"=w141, "ModelEditInfo in"=w143) -> ("ModelEditInfo out"=w134:T9)  [unwired: 8 in, 1 out]
      }
      event "Btn_删除点位": Value Change {
        n91 = event-data() -> ()  [unwired: 1 in, 1 out]
        n92 = call "DeleteTestItem.vi"("ModelEditInfo"=w151) -> ("ModelEditInfo out"=w150:T2)
        n93 = call "禁用不供料的托盘-点位表格内不供料托盘背景红色.vi"("引用Cluster"=w149, "ModelEditInfo in"=w150) -> ("ModelEditInfo out"=w148:T9)  [unwired: 8 in, 1 out]
      }
      event "Btn_更新点位信息表": Value Change {
        n94 = event-data() -> ("NewVal"=w156:bool)  [unwired: 1 in]
        n95 = case shown="真" w156 {
          tunnel: w155 -> [w157 w167]
          tunnel: w154 -> [_ w169]
          tunnel: [w157 w158] -> w153
          tunnel: w152 -> [_ w161]
          frame False {
          }
          frame True {
            n96 = Unbundle By Name(w167) -> ("当前产品所有点位信息.点位信息表"=w170:string[][], "当前产品所有点位信息.当前点位序号"=w168:i32, "当前产品信息"=w166:T13)
            n97 = call "锁附点位信息ClusterToTable.vi"("锁附点位信息"=w169, "当前产品信息"=w166) -> ("点位信息表格一行"=w171:string[])  [unwired: 1 in]
            n98 = Replace Array Subset(array=w170, new element=w171, index (row)=w168) -> (w163:string[][])  [unwired: 1 in]
            n99 = Bundle By Name(cluster=w167, "当前产品所有点位信息.点位信息表"=w163, "当前产品所有点位信息.当前点位序号"=w168) -> (w165:T9)
            n100 = call "UpdateSaveData.vi"("ModelEditInfo in"=w165) -> ("ModelEditInfo out"=w164:T2)
            n101 = call "ReadModelInfo.vi"("更新量测项目序号"=FALSE, "ModelEditInfo in"=w164) -> ("ModelEditInfo out"=w159:T2)  [unwired: 1 in]
            n102 = call "显示点位示意图.vi"("ModelEditInfo"=w159, "显示点位动作"=控件-点位示意图动作."更新点位示意图") -> ()  [unwired: 9 in, 1 out]
            n103 = call "禁用不供料的托盘-点位表格内不供料托盘背景红色.vi"("引用Cluster"=w161, "ModelEditInfo in"=w159) -> ("ModelEditInfo out"=w158:T9)  [unwired: 8 in, 1 out]
            n104 = flat-sequence {
              tunnel: w159 -> [_]
              frame #0 {
                n105 = One Button Dialog(message="点位信息表已更新!\n并且已经保存到本机中！" ("消息")) -> ()  [unwired: 1 in, 1 out]
              }
            }
          }
        }
      }
      event "读取CAD文档点位信息": Value Change {
        n106 = event-data() -> ()  [unwired: 1 in, 1 out]
        n107 = call "读取并解码CAD文档坐标.vi"("ModelEditInfo"=w180) -> ("ModelEditInfo 输出"=w177:T2)  [unwired: 10 in]
        n108 = call "UpdateSaveData.vi"("ModelEditInfo in"=w177) -> ("ModelEditInfo out"=w179:T2)
        n109 = call "ReadModelInfo.vi"("更新量测项目序号"=FALSE, "ModelEditInfo in"=w179) -> ("ModelEditInfo out"=w174:T2)  [unwired: 1 in]
        n110 = flat-sequence {
          tunnel: w174 -> [_]
          frame #0 {
            n111 = One Button Dialog(message="点位信息表中\"拍照点坐标CAD图纸XYZ\"3列值已更新!\n并且已经保存到本机中！" ("消息")) -> ()  [unwired: 1 in, 1 out]
          }
        }
        n112 = call "显示点位示意图.vi"("ModelEditInfo"=w174, "显示点位动作"=控件-点位示意图动作."更新点位示意图") -> ()  [unwired: 9 in, 1 out]
        n113 = call "禁用不供料的托盘-点位表格内不供料托盘背景红色.vi"("引用Cluster"=w176, "ModelEditInfo in"=w174) -> ("ModelEditInfo out"=w173:T9)  [unwired: 8 in, 1 out]
      }
      event "Btn_读取Mark1&Mark2(P21 P22)坐标": Value Change {
        n114 = event-data() -> ("NewVal"=w183:bool)  [unwired: 1 in]
        n115 = case shown="真" w183 {
          tunnel: w184 -> [w185 w190]
          tunnel: [w185 w191] -> w182
          frame False {
          }
          frame True {
            n116 = call "欧姆龙PLC通讯Main-UDP.vi"("欧姆龙PLC Action"=欧姆龙PLC_Action."读第1组Mark点坐标") -> (2:w192, "PLC连线成功"=w186:bool)  [unwired: 7 in, 2 out]
            n117 = case shown="真" w186 {
              tunnel: w192 -> [_ w201]
              tunnel: [w194 w200] -> w191
              tunnel: w190 -> [w194 w199]
              frame False {
              }
              frame True {
                n118 = Unbundle By Name(w201) -> ("PCB1-Mark拍照点坐标"=w195)
                "Mark拍照点坐标" <- w195
                n119 = Unbundle By Name(w199) -> ("Mark拍照点坐标"=w198:T4[][])
                n120 = Replace Array Subset(array=w198, new element=w195, index (row)=0 ("索引")) -> (w197:T4[][])  [unwired: 1 in]
                n121 = Bundle By Name(cluster=w199, "Mark拍照点坐标"=w197) -> (w200:T9)
              }
            }
            n122 = Select(t="从PLC中读取第一组Mark点坐标成功!" ("消息"), s=w186, f="从PLC中读取第一组Mark点坐标失败!\n请检查电脑与PLC交换机之间的连接!" ("消息")) -> (s? t:f=w188:string)
            n123 = One Button Dialog(message=w188) -> ()  [unwired: 1 in, 1 out]
          }
        }
      }
      event #10 (no event record) {
        n124 = event-data() -> ("NewVal"=w204)  [unwired: 1 in]
        n125 = case shown="真" w204 {
          tunnel: w203 -> [w205 w210]
          tunnel: [w205 w211] -> w202
          frame False {
          }
          frame True {
            n126 = call "欧姆龙PLC通讯Main-UDP.vi"("欧姆龙PLC Action"=欧姆龙PLC_Action."读第2组Mark点坐标") -> (2:w212, "PLC连线成功"=w206:bool)  [unwired: 7 in, 2 out]
            n127 = case shown="真" w206 {
              tunnel: w212 -> [_ w221]
              tunnel: [w214 w220] -> w211
              tunnel: w210 -> [w214 w219]
              frame False {
              }
              frame True {
                n128 = Unbundle By Name(w221) -> ("PCB2-Mark拍照点坐标"=w215)
                n129 = Unbundle By Name(w219) -> ("Mark拍照点坐标"=w218:T4[][])
                n130 = Replace Array Subset(array=w218, new element=w215, index (row)=1 ("索引")) -> (w217:T4[][])  [unwired: 1 in]
                n131 = local write "Mark拍照点坐标"(w215) -> ()
                n132 = Bundle By Name(cluster=w219, "Mark拍照点坐标"=w217) -> (w220:T9)
              }
            }
            n133 = Select(t="从PLC中读取第一组Mark点坐标成功!" ("消息"), s=w206, f="从PLC中读取第一组Mark点坐标失败!\n请检查电脑与PLC交换机之间的连接!" ("消息")) -> (s? t:f=w208:string)
            n134 = One Button Dialog(message=w208) -> ()  [unwired: 1 in, 1 out]
          }
        }
      }
      event #11 (no event record) {
        n135 = event-data() -> ("NewVal"=w223)  [unwired: 1 in]
        n136 = case shown="真" w223 {
          tunnel: w224 -> [w225 w230]
          tunnel: [w225 w231] -> w222
          frame False {
          }
          frame True {
            n137 = call "欧姆龙PLC通讯Main-UDP.vi"("欧姆龙PLC Action"=欧姆龙PLC_Action."读第3组Mark点坐标") -> (2:w232, "PLC连线成功"=w226:bool)  [unwired: 7 in, 2 out]
            n138 = case shown="假" w226 {
              tunnel: w232 -> [_ w241]
              tunnel: [w234 w240] -> w231
              tunnel: w230 -> [w234 w239]
              frame False {
              }
              frame True {
                n139 = Unbundle By Name(w241) -> ("PCB3-Mark拍照点坐标"=w235)
                n140 = Unbundle By Name(w239) -> ("Mark拍照点坐标"=w238:T4[][])
                n141 = Replace Array Subset(array=w238, new element=w235, index (row)=2 ("索引")) -> (w237:T4[][])  [unwired: 1 in]
                n142 = local write "Mark拍照点坐标"(w235) -> ()
                n143 = Bundle By Name(cluster=w239, "Mark拍照点坐标"=w237) -> (w240:T9)
              }
            }
            n144 = Select(t="从PLC中读取第一组Mark点坐标成功!" ("消息"), s=w226, f="从PLC中读取第一组Mark点坐标失败!\n请检查电脑与PLC交换机之间的连接!" ("消息")) -> (s? t:f=w228:string)
            n145 = One Button Dialog(message=w228) -> ()  [unwired: 1 in, 1 out]
          }
        }
      }
      event #12 (no event record) {
        n146 = event-data() -> ("NewVal"=w243)  [unwired: 1 in]
        n147 = case shown="真" w243 {
          tunnel: w244 -> [w245 w250]
          tunnel: [w245 w251] -> w242
          frame False {
          }
          frame True {
            n148 = call "欧姆龙PLC通讯Main-UDP.vi"("欧姆龙PLC Action"=欧姆龙PLC_Action."读第4组Mark点坐标") -> (2:w252, "PLC连线成功"=w246:bool)  [unwired: 7 in, 2 out]
            n149 = case shown="假" w246 {
              tunnel: w252 -> [_ w261]
              tunnel: [w254 w260] -> w251
              tunnel: w250 -> [w254 w259]
              frame False {
              }
              frame True {
                n150 = Unbundle By Name(w261) -> ("PCB4-Mark拍照点坐标"=w255)
                n151 = Unbundle By Name(w259) -> ("Mark拍照点坐标"=w258:T4[][])
                n152 = Replace Array Subset(array=w258, new element=w255, index (row)=3 ("索引")) -> (w257:T4[][])  [unwired: 1 in]
                n153 = local write "Mark拍照点坐标"(w255) -> ()
                n154 = Bundle By Name(cluster=w259, "Mark拍照点坐标"=w257) -> (w260:T9)
              }
            }
            n155 = Select(t="从PLC中读取第一组Mark点坐标成功!" ("消息"), s=w246, f="从PLC中读取第一组Mark点坐标失败!\n请检查电脑与PLC交换机之间的连接!" ("消息")) -> (s? t:f=w248:string)
            n156 = One Button Dialog(message=w248) -> ()  [unwired: 1 in, 1 out]
          }
        }
      }
      event "Btn_根据第1组Mark点计算PCB1其它拍照点坐标": Value Change {
        n157 = event-data() -> ()  [unwired: 1 in, 1 out]
        n158 = call "根据两个示教点计算其它点位坐标.vi"("选择计算拍照点的PCB"=T18."计算PCB1其它拍照点坐标", "ModelEditInfo输入"=w270) -> ("ModelEditInfo输出"=w267:T2)  [unwired: 9 in]
        n159 = call "UpdateSaveData.vi"("ModelEditInfo in"=w267) -> ("ModelEditInfo out"=w269:T2)
        n160 = call "ReadModelInfo.vi"("更新量测项目序号"=FALSE, "ModelEditInfo in"=w269) -> ("ModelEditInfo out"=w263:T2)  [unwired: 1 in]
        n161 = call "禁用不供料的托盘-点位表格内不供料托盘背景红色.vi"("引用Cluster"=w265, "ModelEditInfo in"=w263) -> ("ModelEditInfo out"=w262:T9)  [unwired: 8 in, 1 out]
        n162 = call "显示点位示意图.vi"("ModelEditInfo"=w263, "显示点位动作"=控件-点位示意图动作."更新点位示意图") -> ()  [unwired: 9 in, 1 out]
        n163 = flat-sequence {
          tunnel: w263 -> [_]
          frame #0 {
            n164 = One Button Dialog(message="点位信息表中PCB1的点位已更新!\n并且已经保存到本机中！" ("消息")) -> ()  [unwired: 1 in, 1 out]
          }
        }
      }
      event #14 (no event record) {
        n165 = event-data() -> ()  [unwired: 1 in, 1 out]
        n166 = call "根据两个示教点计算其它点位坐标.vi"("选择计算拍照点的PCB"=T18."计算PCB2其它拍照点坐标", "ModelEditInfo输入"=w278) -> ("ModelEditInfo输出"=w273:T2)  [unwired: 9 in]
        n167 = call "UpdateSaveData.vi"("ModelEditInfo in"=w273) -> ("ModelEditInfo out"=w280:T2)
        n168 = call "ReadModelInfo.vi"("更新量测项目序号"=FALSE, "ModelEditInfo in"=w280) -> ("ModelEditInfo out"=w277:T2)  [unwired: 1 in]
        n169 = call "禁用不供料的托盘-点位表格内不供料托盘背景红色.vi"("引用Cluster"=w275, "ModelEditInfo in"=w277) -> ("ModelEditInfo out"=w272:T9)  [unwired: 8 in, 1 out]
        n170 = call "显示点位示意图.vi"("ModelEditInfo"=w273, "显示点位动作"=控件-点位示意图动作."更新点位示意图") -> ()  [unwired: 9 in, 1 out]
        n171 = flat-sequence {
          tunnel: w273 -> [_]
          frame #0 {
            n172 = One Button Dialog(message="点位信息表中PCB2的点位已更新!\n并且已经保存到本机中！" ("消息")) -> ()  [unwired: 1 in, 1 out]
          }
        }
      }
      event #15 (no event record) {
        n173 = event-data() -> ()  [unwired: 1 in, 1 out]
        n174 = call "根据两个示教点计算其它点位坐标.vi"("选择计算拍照点的PCB"=T18."计算PCB3其它拍照点坐标", "ModelEditInfo输入"=w288) -> ("ModelEditInfo输出"=w284:T2)  [unwired: 9 in]
        n175 = call "UpdateSaveData.vi"("ModelEditInfo in"=w284) -> ("ModelEditInfo out"=w290:T2)
        n176 = call "ReadModelInfo.vi"("更新量测项目序号"=FALSE, "ModelEditInfo in"=w290) -> ("ModelEditInfo out"=w282:T2)  [unwired: 1 in]
        n177 = call "禁用不供料的托盘-点位表格内不供料托盘背景红色.vi"("引用Cluster"=w286, "ModelEditInfo in"=w282) -> ("ModelEditInfo out"=w283:T9)  [unwired: 8 in, 1 out]
        n178 = call "显示点位示意图.vi"("ModelEditInfo"=w282, "显示点位动作"=控件-点位示意图动作."更新点位示意图") -> ()  [unwired: 9 in, 1 out]
        n179 = flat-sequence {
          tunnel: w283 -> [_]
          frame #0 {
            n180 = One Button Dialog(message="点位信息表中PCB3的点位已更新!\n并且已经保存到本机中！" ("消息")) -> ()  [unwired: 1 in, 1 out]
          }
        }
      }
      event #16 (no event record) {
        n181 = event-data() -> ()  [unwired: 1 in, 1 out]
        n182 = call "根据两个示教点计算其它点位坐标.vi"("选择计算拍照点的PCB"=T18."计算PCB4其它拍照点坐标", "ModelEditInfo输入"=w298) -> ("ModelEditInfo输出"=w294:T2)  [unwired: 9 in]
        n183 = call "UpdateSaveData.vi"("ModelEditInfo in"=w294) -> ("ModelEditInfo out"=w300:T2)
        n184 = call "ReadModelInfo.vi"("更新量测项目序号"=FALSE, "ModelEditInfo in"=w300) -> ("ModelEditInfo out"=w293:T2)  [unwired: 1 in]
        n185 = call "禁用不供料的托盘-点位表格内不供料托盘背景红色.vi"("引用Cluster"=w296, "ModelEditInfo in"=w293) -> ("ModelEditInfo out"=w292:T9)  [unwired: 8 in, 1 out]
        n186 = call "显示点位示意图.vi"("ModelEditInfo"=w293, "显示点位动作"=控件-点位示意图动作."更新点位示意图") -> ()  [unwired: 9 in, 1 out]
        n187 = flat-sequence {
          tunnel: w292 -> [_]
          frame #0 {
            n188 = One Button Dialog(message="点位信息表中PCB4的点位已更新!\n并且已经保存到本机中！" ("消息")) -> ()  [unwired: 1 in, 1 out]
          }
        }
      }
      event "Btn_PCB2~4锁螺丝时机械手角度，取料托盘号与PCB1相同": Value Change {
        # "每次更新点位信息，这一步强制执行，所以去掉此按钮事件"
        n189 = event-data() -> ()  [unwired: 1 in, 1 out]
        n190 = call "PCB234锁螺丝时机械手角度-取料托盘号与PCB1相同.vi"("ModelEditInfo输入"=w308) -> ("ModelEditInfo out"=w303:T9)  [unwired: 9 in, 1 out]
        n191 = call "UpdateSaveData.vi"("ModelEditInfo in"=w303) -> ("ModelEditInfo out"=w307:T2)
        n192 = call "ReadModelInfo.vi"("更新量测项目序号"=FALSE, "ModelEditInfo in"=w307) -> ("ModelEditInfo out"=w305:T2)  [unwired: 1 in]
        n193 = call "禁用不供料的托盘-点位表格内不供料托盘背景红色.vi"("引用Cluster"=w304, "ModelEditInfo in"=w305) -> ("ModelEditInfo out"=w302:T9)  [unwired: 8 in, 1 out]
        n194 = flat-sequence {
          tunnel: w302 -> [_]
          frame #0 {
            n195 = One Button Dialog(message="点位信息表中其它PCB的锁螺丝角度，取料托盘等信息已更新与PCB1一致!\n并且已经保存到本机中！" ("消息")) -> ()  [unwired: 1 in, 1 out]
          }
        }
      }
      event #18 (no event record) {
        n196 = event-data() -> ("CtlRef"=w313, "Double Click"=w312)  [unwired: 1 in]
        n197 = Unbundle By Name(w315) -> ("当前产品所有点位信息.点位信息表"=w323:string[][], "当前产品信息"=w311:T13)
        n198 = property class="Tbl (严格)"(reference=w313) -> ("EditPos"=w316:T19)  [unwired: 1 in, 2 out]
        n199 = Array Size(array=w323) -> (size(s)=w319:i32[])
        n200 = Unbundle By Name(w316) -> ("Row"=w322:i32)
        n201 = Index Array(array=w319) -> (element=w320:i32)  [unwired: 1 in]
        n202 = Less?(x=w322, y=w320) -> (x < y?=w317:bool)
        n203 = Greater Or Equal To 0?(x=w322) -> (x >= 0?=w318:bool)
        n204 = And(x=w317, y=w318) -> (x .and. y?=w321:bool)
        n205 = case shown="真" w321 {
          tunnel: w322 -> [_ w330]
          tunnel: w323 -> [_ w332]
          tunnel: w312 -> [_ w331]
          tunnel: w315 -> [w324 w329]
          tunnel: [w324 w326] -> w314
          tunnel: w311 -> [_ w327]
          tunnel: w310 -> [_ w325]
          frame False {
          }
          frame True {
            n206 = case shown="真" w331 {
              tunnel: w332 -> [_ w339]
              tunnel: w330 -> [_ w338]
              tunnel: w329 -> [w333 w337]
              tunnel: [w333 w336] -> w328
              tunnel: w327 -> [_ w334]
              frame False {
              }
              frame True {
                n207 = call "点位信息表ToCluster.vi"("Row"=w338, "当前产品信息"=w334, "锁附点位信息表"=w339) -> ("锁附点位信息"=w335:T10)
                n208 = Bundle By Name(cluster=w337, "当前产品所有点位信息.当前点位信息"=w335) -> (w336:T9)
              }
            }
            n209 = Bundle By Name(cluster=w328, "当前产品所有点位信息.当前点位序号"=w330) -> (w326:T9)
            n210 = call "禁用不供料的托盘-点位表格内不供料托盘背景红色.vi"("引用Cluster"=w325, "ModelEditInfo in"=w326) -> ()  [unwired: 8 in, 2 out]
          }
        }
      }
      event "Btn_更新拧紧程式参数": Value Change {
        n211 = event-data() -> ("NewVal"=w347:bool)  [unwired: 1 in]
        n212 = control-ref of="拧紧程式参数表"() -> (w343:refnum<vi>)
        n213 = call "检查拧紧程式.vi"("拧紧程式参数表引用"=w343, "拧紧程式参数表输入"=w342, "ModelEditInfo"=w341) -> ("异常显示信息"=w344:string, "拧紧程式参数表设定OK"=w340:bool)  [unwired: 7 in]
        n214 = case shown="真" w340 {
          tunnel: w347 -> [_ w356]
          tunnel: w342 -> [_ w355]
          tunnel: w341 -> [w350 w354]
          tunnel: [w350 w353] -> w346
          tunnel: w345 -> [_ w352]
          tunnel: w344 -> [w348 _]
          frame False {
            n215 = local write "Btn_更新拧紧程式参数"(FALSE ("Btn_更新拧紧程式参数")) -> ()
            n216 = One Button Dialog(message=w348) -> ()  [unwired: 1 in, 1 out]
          }
          frame True {
            n217 = case shown="真" w356 {
              tunnel: w355 -> [_ w364]
              tunnel: w354 -> [w357 w365]
              tunnel: [w357 w358] -> w353
              tunnel: w352 -> [_ w359]
              frame False {
              }
              frame True {
                n218 = Bundle By Name(cluster=w365, "拧紧程式参数.所有拧紧程式参数表"=w364) -> (w363:T9)
                n219 = call "保存拧紧程式参数表.vi"("ModelEditInfo in"=w363) -> ("写表格结果"=w361:bool, "ModelEditInfo out"=w362:T9)  [unwired: 9 in]
                n220 = case shown="假" w361 {
                  tunnel: [w370 w371] -> w360
                  tunnel: w362 -> [w370 w371]
                  frame False {
                    n221 = Unbundle By Name(w370) -> ("拧紧程式参数.所有拧紧程式参数表"=w369:string[][])
                    n222 = local write "拧紧程式参数表"(w369) -> ()
                  }
                  frame True {
                  }
                }
                n223 = Select(t="拧紧程式参数表已更新!\n并且已经保存到本机中！" ("消息"), s=w361, f="拧紧程式参数表更新失败!" ("消息")) -> (s? t:f=w367:string)
                n224 = One Button Dialog(message=w367) -> ()  [unwired: 1 in, 1 out]
                n225 = call "禁用不供料的托盘-点位表格内不供料托盘背景红色.vi"("引用Cluster"=w359, "ModelEditInfo in"=w360) -> ("ModelEditInfo out"=w358:T9)  [unwired: 8 in, 1 out]
              }
            }
            n226 = local write "Btn_更新拧紧程式参数"(FALSE ("Btn_更新拧紧程式参数")) -> ()
          }
        }
      }
      event "Btn_删除拧紧程式参数": Value Change {
        n227 = event-data() -> ()  [unwired: 1 in, 1 out]
        n228 = call "删除拧紧程式参数表的某一行.vi"("ModelEditInfo"=w379) -> ("ModelEditInfo out"=w378:T9)  [unwired: 1 in]
        n229 = Unbundle By Name(w378) -> ("拧紧程式参数.所有拧紧程式参数表"=w377:string[][], "拧紧程式参数.所有拧紧程式参数表当前行"=w375:i32)
        n230 = control-ref of="拧紧程式参数表"() -> (w376:refnum<vi>)
        n231 = flat-sequence {
          tunnel: w378 -> [w381]
          tunnel: [w381] -> w374
          frame #0 {
            n232 = local write "Btn_删除拧紧程式参数"(FALSE ("Btn_删除拧紧程式参数")) -> ()
          }
        }
        n233 = local write "拧紧程式参数表"(w377) -> ()
        n234 = call "高亮当前行.vi"("Row"=w375, "Table输入"=w376) -> ()  [unwired: 9 in, 1 out]
        n235 = call "禁用不供料的托盘-点位表格内不供料托盘背景红色.vi"("引用Cluster"=w372, "ModelEditInfo in"=w374) -> ("ModelEditInfo out"=w373:T9)  [unwired: 8 in, 1 out]
      }
      event "拧紧程式参数表": Mouse Up {
        n236 = event-data() -> ("CtlRef"=w385:refnum<vi>, "Mods.Double Click"=w384:bool)  [unwired: 1 in]
        n237 = Unbundle By Name(w383) -> ("拧紧程式参数.所有拧紧程式参数表"=w382:string[][])
        n238 = property class="Tbl (严格)"(reference=w385) -> ("EditPos"=w387:T19)  [unwired: 1 in, 2 out]
        n239 = Array Size(array=w382) -> (size(s)=w390:i32[])
        n240 = Unbundle By Name(w387) -> ("Row"=w393:i32)
        n241 = Index Array(array=w390) -> (element=w391:i32)  [unwired: 1 in]
        n242 = Less?(x=w393, y=w391) -> (x < y?=w388:bool)
        n243 = Greater Or Equal To 0?(x=w393) -> (x >= 0?=w389:bool)
        n244 = And(x=w388, y=w389) -> (x .and. y?=w392:bool)
        n245 = case shown="真" w392 {
          tunnel: w393 -> [_ w399]
          tunnel: w384 -> [_ _]
          tunnel: w383 -> [w394 w396]
          tunnel: [w394 w395] -> w386
          tunnel: w382 -> [_ w397]
          frame False {
          }
          frame True {
            n246 = Bundle By Name(cluster=w396, "拧紧程式参数.所有拧紧程式参数表当前行"=w399) -> (w395:T9)
            n247 = control-ref of="拧紧程式参数表"() -> (w398:refnum<vi>)
            n248 = call "检查拧紧程式.vi"("拧紧程式参数表引用"=w398, "拧紧程式参数表输入"=w397, "ModelEditInfo"=w395) -> ()  [unwired: 7 in, 2 out]
          }
        }
      }
      event "退出按钮": Value Change {
        n249 = event-data() -> ("NewVal"=w402:bool)  [unwired: 1 in]
        n250 = case shown="真" w402 {
          tunnel: w400 -> [_ w408]
          tunnel: [FALSE w409] -> w401
          frame False {
          }
          frame True {
            n251 = Unbundle By Name(w408) -> ("已勾选的自动锁螺丝点位供料盘设定错误"=w407:bool, "已勾选的自动锁螺丝点位拧紧程式序号设定错误"=w406:bool)
            n252 = Or(x=w407, y=w406) -> (x .or. y?=w405:bool)
            n253 = case shown="真" w405 {
              tunnel: [w411 w420] -> w409
              tunnel: w408 -> [w410 _]
              frame False {
                n254 = flat-sequence {
                  tunnel: w410 -> [w417]
                  tunnel: [TRUE] -> w411
                  frame #0 {
                    n255 = Unbundle By Name(w417) -> ("AllModelFold"=w416:path, "当前零件序号"=w413:i32)
                    n256 = Build Array(w413) -> (w418:i32[])
                    n257 = Build Path(base path=w416, name or relative path="CurrentModelNameIndex.txt") -> (appended path=w415:path)
                    n258 = call-poly <vilib>:"Write To Spreadsheet File.vi"("append to file? (new file:F)"=FALSE, "1D data"=w418, "file path (dialog if empty)"=w415) -> ()  [unwired: 5 in, 1 out]
                  }
                  frame #1 {
                  }
                }
              }
              frame True {
                n259 = Two Button Dialog(message="某些点位(红色背景)选择的供料盘没有供料(没有选择螺丝型号)，\n或者选择的拧紧程式序号还未设定参数(拧紧程式参数表中不存在该序号)，\n请重新维护相应参数，或者该点位选择不自动锁后，再退出！" ("消息"), 1:"强制退出维护页面" ("F按钮名称（“取消”）"), 2:"不退出，继续维护参数" ("T按钮名称（“确定”）")) -> (T button?=w421:bool)
                n260 = Not(x=w421) -> (.not. x?=w420:bool)
              }
            }
            n261 = Not(x=w405) -> (.not. x?=→"产品程式设定OK":bool)
          }
        }
      }
    }
    n262 = Wait Until Next ms Multiple(millisecond multiple=u32 50) -> ()  [unwired: 1 out]
    n263 = local write "ModelEditInfo"(w36) -> ()
  }
  "ModelEditInfo" <- w33
  n264 = Array Subset(array=w9, index=1 ("索引")) -> (w7:string[])  [unwired: 1 in]
  n265 = Build Array(w7) -> (w6:string[][])
  n266 = Transpose 2D Array(2D array=w6) -> (transposed array=→"不同型号螺丝放料点与拍照点高度差":string[][])
